vi "Shake Tray.vi"(8 "error in (no error)":errorcluster, 11 "Autosampler in":refnum<class "Autosampler.lvclass">) -> (0 "error out":errorcluster, 3 "Autosampler out":refnum<class "Autosampler.lvclass">)   [LabVIEW 2023, in "Autosampler.lvlib" / "Autosampler.lvclass"]
uses:
  Autosampler.lvclass
  Autosampler State2.ctl
  Autosampler.lvclass/Autosampler.ctl
  Autosampler.lvlib
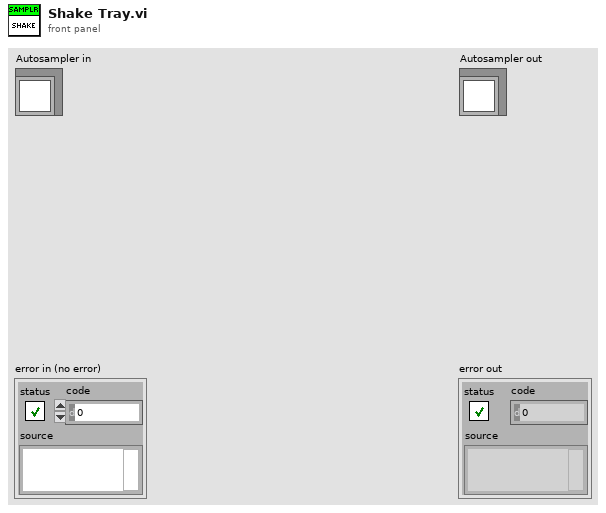
[diagram p1: front panel]
types:
  T1 = typedef "Autosampler.lvlib/Autosampler State2.ctl" = enum16{"Error", "Idle", "Positioning", "Pumping", "Shaking", "Washing", "Priming"}
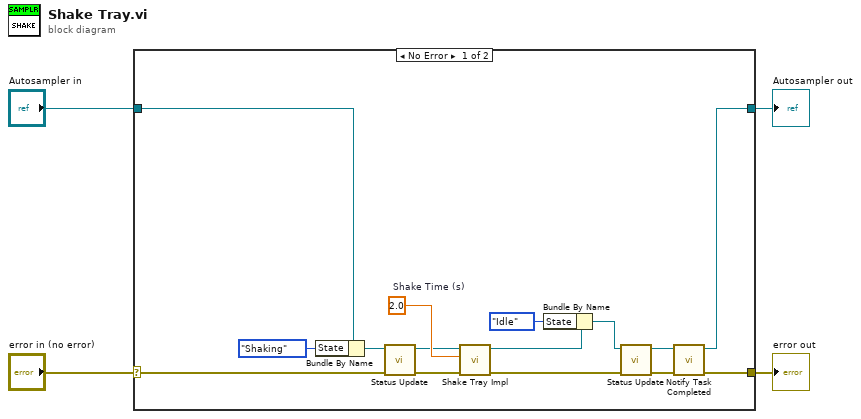
[diagram p0: block diagram]
diagram:
  n1 = case shown="No Error" "error in (no error)" {
    selector: "error in (no error)" -> [w14 w21]
    tunnel: [w18 w21] -> w3
    tunnel: [w17 w20] -> w1
    tunnel: "Autosampler in" -> [w12 w20]
    frame No Error {
      w19 = 2.0  # Shake Time (s)
      n2 = Bundle By Name(cluster=w12, "State"=Autosampler_State2."Shaking") -> (w15:refnum<class "Autosampler.lvclass">)
      n3 = call "Status Update.vi"("error in (no error)"=w14, "Autosampler in"=w15) -> ("error out"=w13:errorcluster, "Autosampler out"=w11:refnum<class "Autosampler.lvclass">)  [unwired: 7 in, 1 out]
      n4 = call-dynamic "Shake Tray Impl.vi"("error in (no error)"=w13, "Time (s)"=w19, "Autosampler in"=w11) -> ("error out"=w10:errorcluster, "Autosampler out"=w6:refnum<class "Autosampler.lvclass">)  [unwired: 7 in]
      n5 = Bundle By Name(cluster=w6, "State"=Autosampler_State2."Idle") -> (w5:refnum<class "Autosampler.lvclass">)
      n6 = call "Status Update.vi"("error in (no error)"=w10, "Autosampler in"=w5) -> ("error out"=w9:errorcluster, "Autosampler out"=w8:refnum<class "Autosampler.lvclass">)  [unwired: 7 in, 1 out]
      n7 = call-dynamic "Notify Task Completed.vi"("error in (no error)"=w9, "Device in"=w8) -> ("error out"=w18:errorcluster, "Device out"=w17:refnum<class "Autosampler.lvclass">)  [unwired: 8 in]
    }
    frame Error {
    }
  }
  "error out" <- w3
  "Autosampler out" <- w1
